vi "Get Document.vi"(8 "error in (no error)":errorcluster caption="entrée d'erreur (pas d'erreur)", 11 "Firebase (Default) en entrée":refnum<class "Firebase Driver.lvclass">) -> (0 "error out":errorcluster caption="sortie d'erreur", 3 "Firebase (Default) en sortie":refnum<class "Firebase Driver.lvclass">)   [LabVIEW 2020, in "Library Instrument & Equipement.lvlib" / "Library FireBase.lvlib" / "Firebase Driver.lvclass"]
uses:
  Firebase Driver.lvclass
  Commun VI/TypeDef/Liste Error.ctl
  Firebase Driver.lvclass/Firebase Driver.ctl
  <vilib>/httpClient/LabVIEWHTTPClient.lvlib
  Commun VI/Library Commun.lvlib
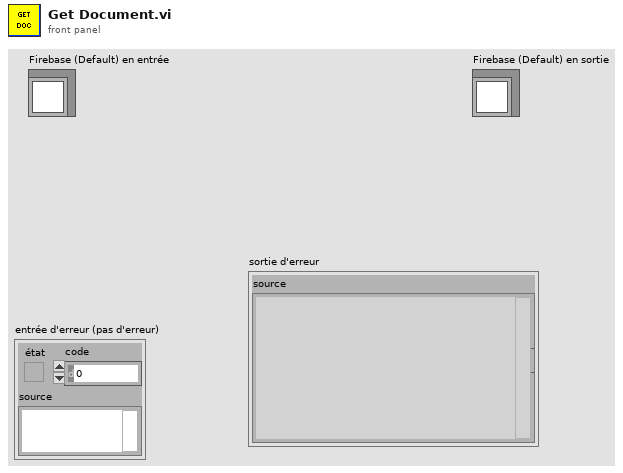
[diagram p1: front panel]
types:
  T1 = typedef "Library Commun.lvlib/Liste Error.ctl" = enum16{"Firebase Driver - Get Document", "Firebase Driver - Get Document With Where", "Firebase Driver - Delete Document", "Firebase Driver - Set Document", "Firebase Driver - Update Document", "Firebase Altyor - Search Document Bench", "Firebase Altyor - Class Not in Firebase", "Spectrum_Analyser - Timeout", "Relay Board - Qty Relay", "DIO - Pb Funtion", "Power_Supply - Peripherical not find", "Mutimeter - Peripherical not find", "Instrument - Function Not Used", "Instrument - Instrument name not specified", "Instrument - Allready Initialised", "Instrument - TimeOut", "Instrument - the instrument must be Initialise before", "Instrument - Frame Not received", "Instrument - Frame Nok", "Test - Initialise the File_for_Save", "Test - Timeout", "Test - Cmd Error", "FGV - Variable ", "BDD FireBase - Define Class", "SN - Class Not Define"}
  T2 = typedef "LabVIEWHTTPClient.lvlib/ClientHandle.ctl" = refnum<k1>
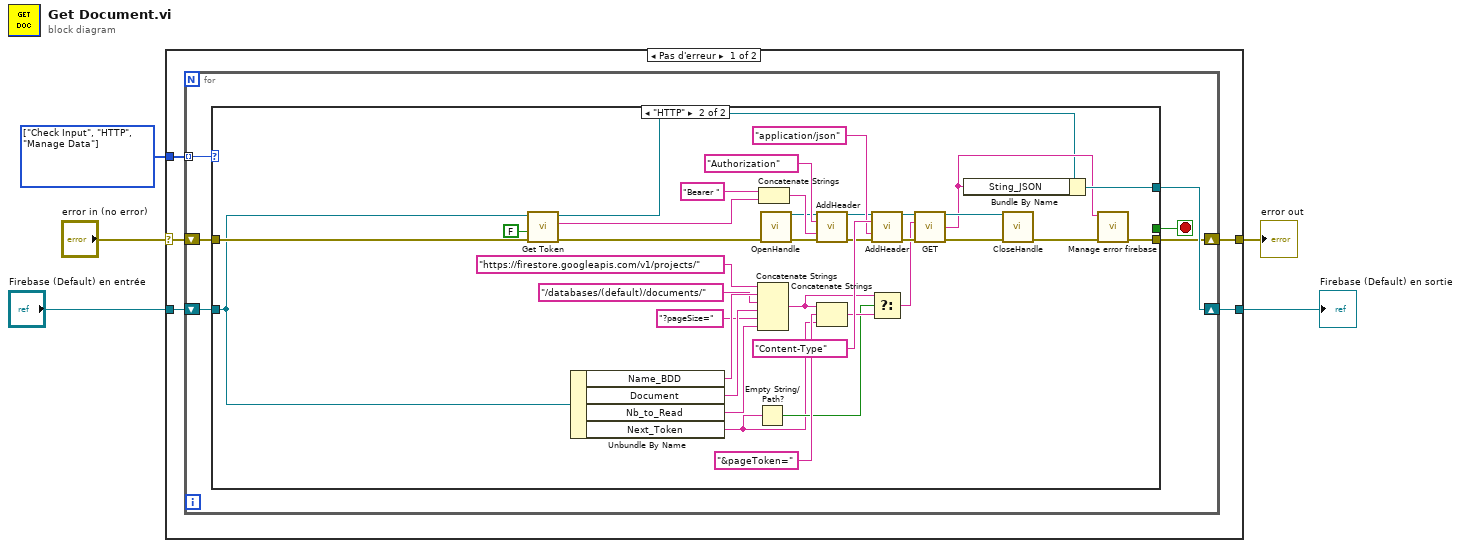
[diagram p0: block diagram]
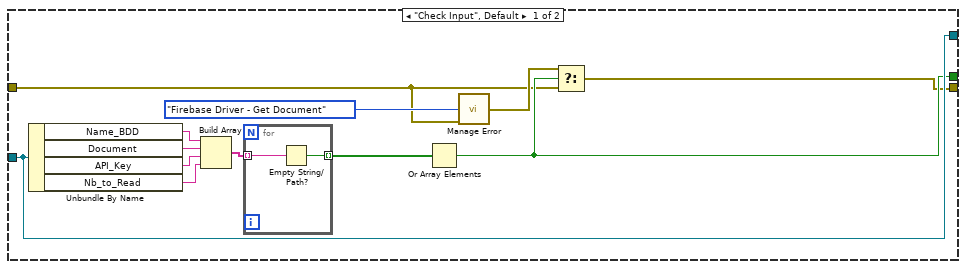
[diagram p2: hidden frame]
diagram:
  w1 = enum16{"Check Input", "HTTP", "Manage Data"}[] [enum."Check Input", enum."HTTP", enum."Manage Data"] items=["Check Input", "HTTP", "Manage Data"]
  n1 = case shown="Pas d'erreur" "error in (no error)" {
    selector: "error in (no error)" -> [w10 w67]
    tunnel: [w9 w67] -> w4
    tunnel: "Firebase (Default) en entrée" -> [w8 w66]
    tunnel: [w7 w66] -> w2
    tunnel: w1 -> [w6 _]
    frame No Error {
      n2 = for {
        shift-right: [w13] -> w9
        shift-left: w10 -> [w16]
        shift-right: [w14] -> w7
        shift-left: w8 -> [w15]
        tunnel: w6 -> [w12] mode=indexing
        stop <- w11 stop-if-true
        n3 = case shown="\"HTTP\"" w12 {
          tunnel: w16 -> [w17 w65]
          tunnel: w15 -> [w28 w44]
          tunnel: [w28 w48] -> w14
          tunnel: [w22 w49] -> w13
          tunnel: [w23 _] -> w11
          frame "Check Input", Default {
            n4 = Unbundle By Name(w28) -> ("Name_BDD"=w27:string, "Document"=w21:string, "API_Key"=w26:string, "Nb_to_Read"=w20:string)
            n5 = Build Array(w27, w21, w26, w20) -> (w25:string[])
            n6 = for {
              tunnel: w25 -> [w30] mode=indexing
              tunnel: [w29] -> w24 mode=indexing
              n7 = Empty String/Path?(string/path=w30) -> (empty?=w29:bool)
            }
            n8 = Or Array Elements(Boolean array=w24) -> (logical OR=w23:bool)
            n9 = call "Manage Error.vi"("Code Erreur"=Liste_Error."Firebase Driver - Get Document", "error in (no error)"=w17) -> ("error out"=w18:errorcluster)  [unwired: 13 in]
            n10 = Select(t=w18, s=w23, f=w17) -> (s? t:f=w22:errorcluster)
          }
          frame "HTTP" {
            n11 = call-dynamic "Get Token.vi"("error in (no error)"=w65, "Reset"=FALSE, "Build Library FireBase.lvlib:Firebase (Default) IN"=w44) -> ("error out"=w50:errorcluster, "idToken"=w46:string, "Build Library FireBase.lvlib:Firebase (Default) Out"=w45:refnum<class "Firebase Driver.lvclass">)  [unwired: 6 in]
            n12 = Unbundle By Name(w44) -> ("Name_BDD"=w41:string, "Document"=w43:string, "Nb_to_Read"=w38:string, "Next_Token"=w34:string)
            n13 = Empty String/Path?(string/path=w34) -> (empty?=w35:bool)
            n14 = Concatenate Strings("https://firestore.googleapis.com/v1/projects/" ("string"), w41, "/databases/(default)/documents/" ("string"), w43, "?pageSize=" ("chaîne"), w38) -> (w32:string)
            n15 = Concatenate Strings("Bearer " ("chaîne"), w46) -> (w56:string)
            n16 = call <vilib>:"OpenHandle.vi"("error in (no error)"=w50) -> ("client handle out"=w55:T2, "error out"=w53:errorcluster)  [unwired: 13 in]
            n17 = call <vilib>:"AddHeader.vi"("client handle"=w55, "header"="Authorization", "value"=w56, "error in (no error)"=w53) -> ("client handle out"=w59:T2, "error out"=w60:errorcluster)  [unwired: 10 in]
            n18 = Concatenate Strings(w32, "&pageToken=" ("chaîne"), w34) -> (w36:string)
            n19 = call <vilib>:"AddHeader.vi"("client handle"=w59, "header"="Content-Type", "value"="application/json", "error in (no error)"=w60) -> ("client handle out"=w54:T2, "error out"=w52:errorcluster)  [unwired: 10 in]
            n20 = Select(t=w32, s=w35, f=w36) -> (s? t:f=w33:string)
            n21 = call <vilib>:"GET.vi"("client handle"=w54, "url"=w33, "error in (no error)"=w52) -> ("client handle out"=w64:T2, "body"=w47:string, "error out"=w63:errorcluster)  [unwired: 9 in, 1 out]
            n22 = Bundle By Name(cluster=w45, "Sting_JSON"=w47) -> (w48:refnum<class "Firebase Driver.lvclass">)
            n23 = call <vilib>:"CloseHandle.vi"("client handle"=w64, "error in (no error)"=w63) -> ("error out"=w51:errorcluster)  [unwired: 13 in]
            n24 = call "Manage error firebase.vi"("error in (no error)"=w51, "Body"=w47) -> ("error out"=w49:errorcluster)  [unwired: 9 in]
          }
        }
      }
    }
    frame Error {
    }
  }
  "error out" <- w4
  "Firebase (Default) en sortie" <- w2
